vi "WristSlantSendCmd.vi"(8 "error in (no error)":errorcluster) -> (0 "error out":errorcluster)   [LabVIEW 2023]
doc: "Sends a boolean command to the boolean receive called \"WristSlant\" (in WristExecuteLogic.vi) to set the Wrist to Slant position to deposit Coral on L4 (-36 deg, check later)\n\nInputs:\n--error in\nOuputs:\n--error out"
uses:
  <vilib>/Rock Robotics/WPI/ThirdParty/JAS_Junk/TrajLib/VI/BoolCmd_Send_Internal.vi
  <vilib>/Rock Robotics/WPI/ThirdParty/JAS_Junk/TrajLib/VI/BoolCmd_ObtainQueue.vi
  <vilib>/Rock Robotics/WPI/ThirdParty/JAS_Junk/TrajLib/Trajectory_Library.lvlib
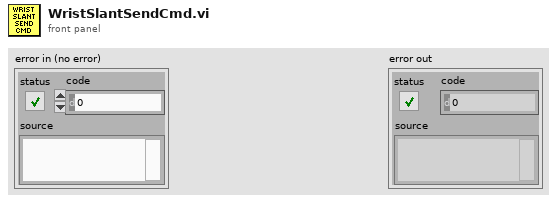
[diagram p1: front panel]
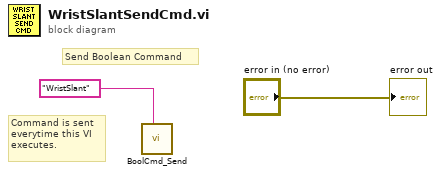
[diagram p0: block diagram]
diagram:
  # "Command is sent\neverytime this VI\nexecutes."
  # "Send Boolean Command"
  n1 = call <vilib>:"BoolCmd_Send.vi"("Command Name"="WristSlant") -> ()  [unwired: 10 in, 1 out]
  "error out" <- "error in (no error)"
